vi "Tree_AddItem.vi"(8 "Error In":errorcluster, 9 "NEW String":string, 10 "Tag at add position":string, 11 "Tree Refnum":refnum<vi>) -> (0 "Error Out":errorcluster, 2 "Added Item Tag":string, 3 "Tree Refnum OUT":refnum<vi>)   [LabVIEW 2012]
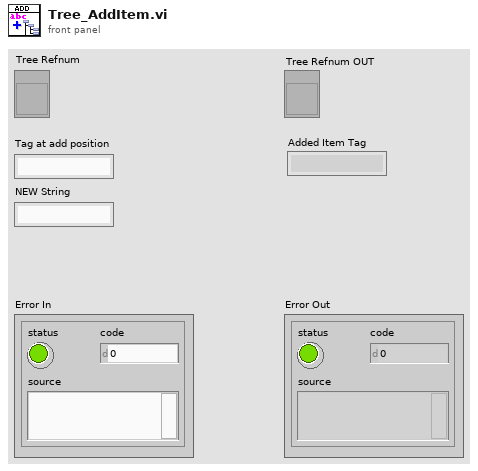
[diagram p1: front panel]
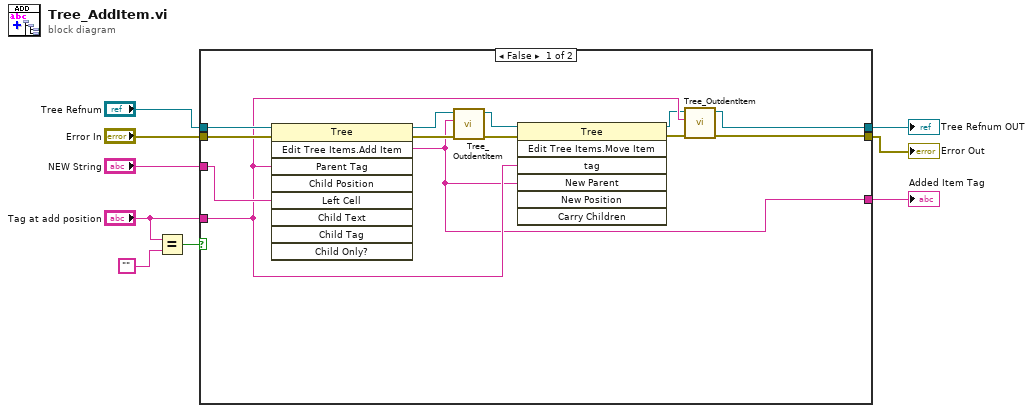
[diagram p0: block diagram]
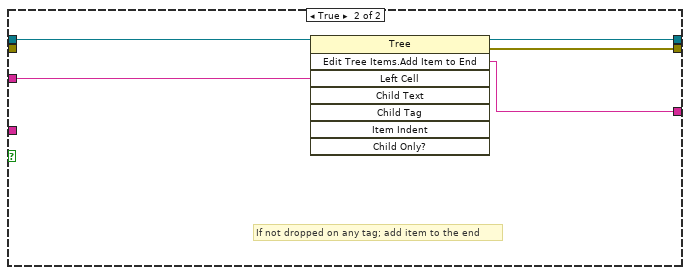
[diagram p2: hidden frame]
diagram:
  n1 = Equal?(x="Tag at add position", y="") -> (x = y?=w8:bool)
  n2 = case shown="False" w8 {
    tunnel: "Tree Refnum" -> [w18 w27]
    tunnel: [w19 w26] -> w6
    tunnel: "Tag at add position" -> [w17 _]
    tunnel: "NEW String" -> [w21 w24]
    tunnel: "Error In" -> [w22 _]
    tunnel: [w20 w25] -> w2
    tunnel: [w10 w23] -> w1
    frame False {
      n3 = invoke class="Tree" method="Edit Tree Items.Add Item"(reference=w18, error in=w22, "Parent Tag"=w17, "Left Cell"=w21) -> (reference out=w12:refnum<vi>, error out=w11:errorcluster, "Edit Tree Items:Add Item"=w10:string)  [unwired: 5 in, 6 out]
      n4 = call "Tree_OutdentItem.vi"("Error In"=w11, "TagToOutdent"=w10, "Tree Refnum"=w12) -> ("Error Out"=w13:errorcluster, "Tree Refnum OUT"=w14:refnum<vi>)  [unwired: 7 in]
      n5 = invoke class="Tree" method="Edit Tree Items.Move Item"(reference=w14, error in=w13, "tag"=w17, "New Parent"=w10) -> (reference out=w15:refnum<vi>, error out=w16:errorcluster)  [unwired: 3 in, 5 out]
      n6 = call "Tree_OutdentItem.vi"("Error In"=w16, "TagToOutdent"=w17, "Tree Refnum"=w15) -> ("Error Out"=w20:errorcluster, "Tree Refnum OUT"=w19:refnum<vi>)  [unwired: 7 in]
    }
    frame True {
      # "If not dropped on any tag; add item to the end"
      n7 = invoke class="Tree" method="Edit Tree Items.Add Item to End"(reference=w27, "Left Cell"=w24) -> (reference out=w26:refnum<vi>, error out=w25:errorcluster, "Edit Tree Items:Add Item to End"=w23:string)  [unwired: 6 in, 5 out]
    }
  }
  "Error Out" <- w2
  "Tree Refnum OUT" <- w6
  "Added Item Tag" <- w1
